vi "Button Grey.vi"(8 "error constant":errorcluster, 9 "Model Name":T1, 10 "appended array 2":bool[](array[boolean]), 11 "appended array":refnum<vi>[](array[refnum])) -> (0 "error constant 2":errorcluster)   [LabVIEW 2017]
uses:
  controls/Model Name.ctl
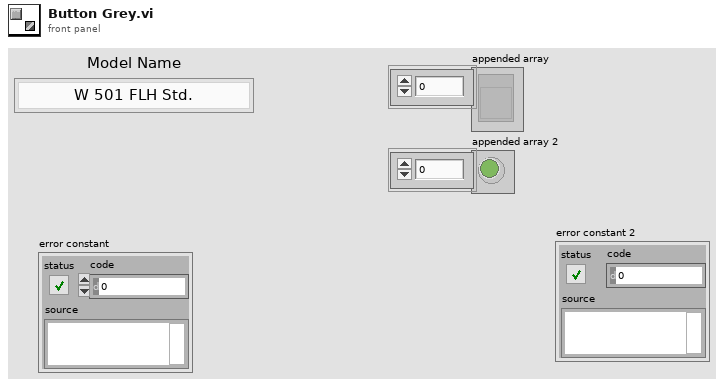
[diagram p1: front panel]
types:
  T1 = typedef "Model Name.ctl" = enum16{"W 501 FLH Std.", "W 501 FRH Std.", "W 601 FR RH Std", "W 601 FR LH Std", "W 601 RR RH Std", "W 601 RR LH Std", "W 601 FR RH AP", "W 601 FR LH AP", "W 601 RR RH AP", "W 601 RR LH AP"}
  T2 = enum8{"Enabled", "Disabled", "Disabled and Grayed Out"}
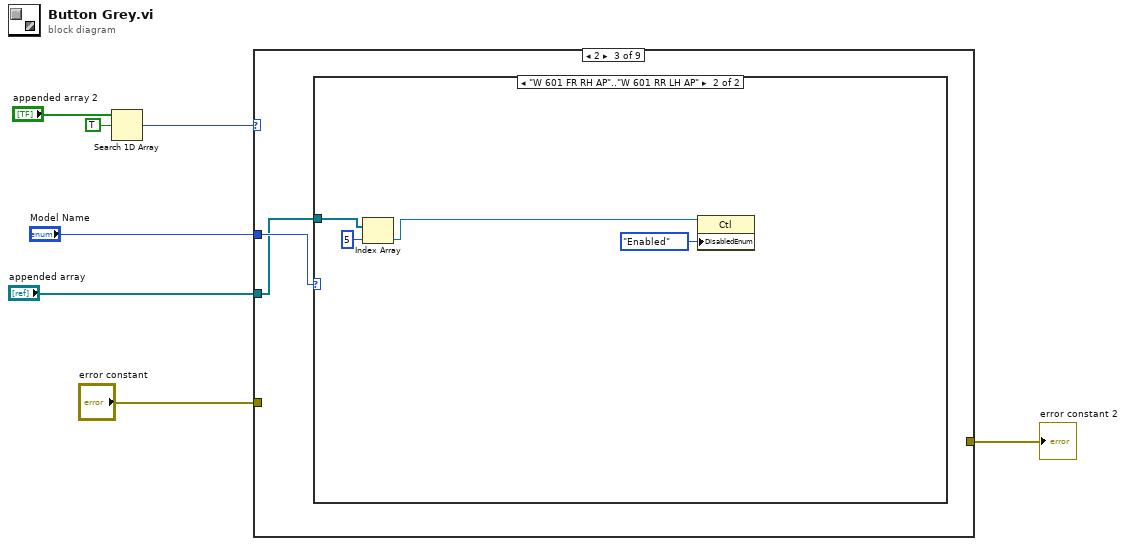
[diagram p0: block diagram]
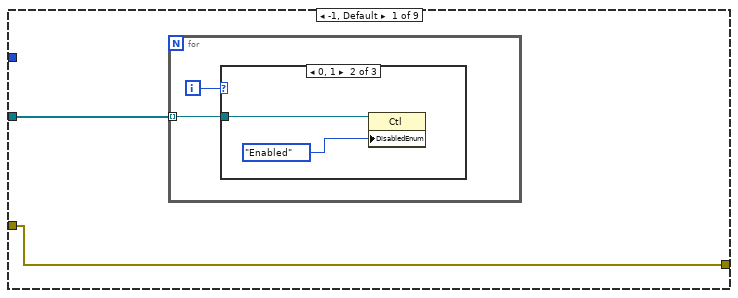
[diagram p2: hidden frame]
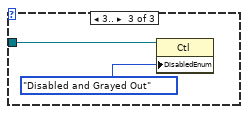
[diagram p4: hidden frame]
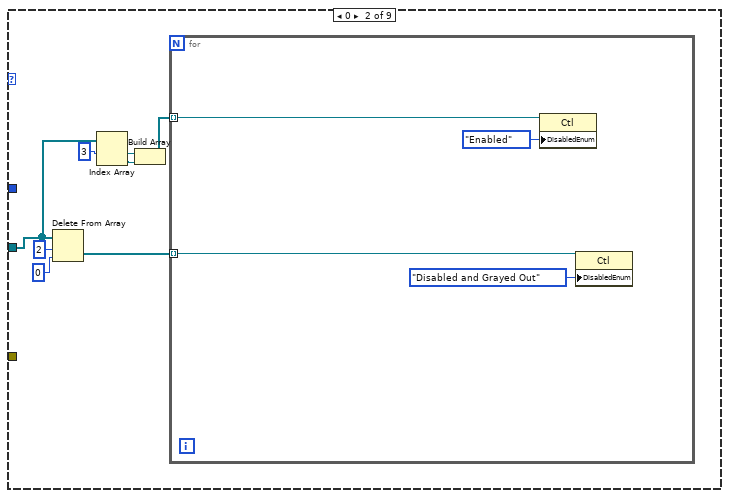
[diagram p5: hidden frame]
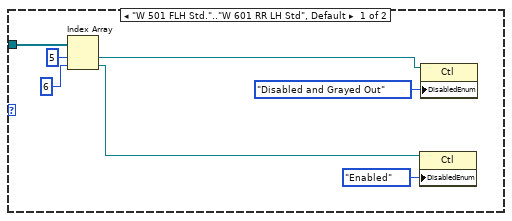
[diagram p6: hidden frame]
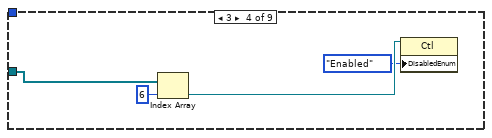
[diagram p7: hidden frame]
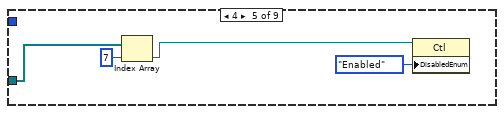
[diagram p8: hidden frame]
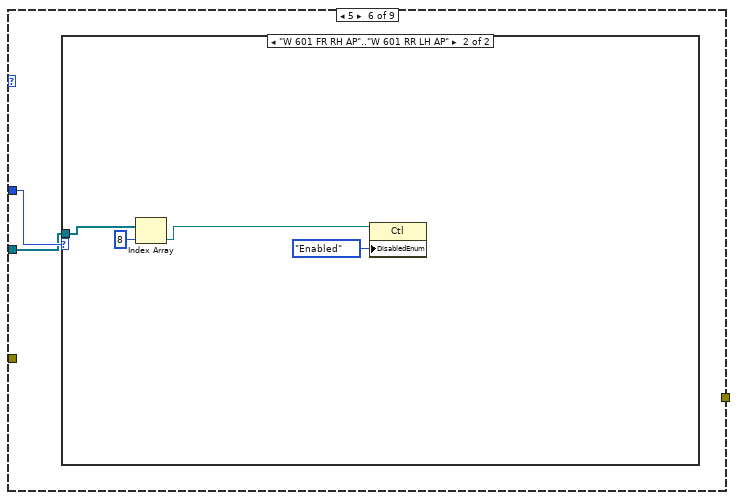
[diagram p9: hidden frame]
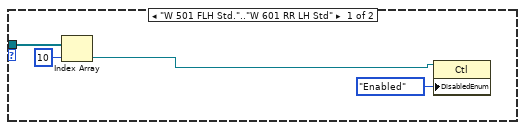
[diagram p10: hidden frame]
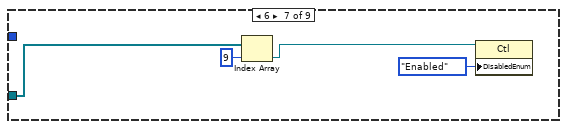
[diagram p11: hidden frame]
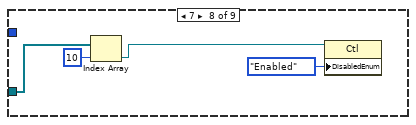
[diagram p12: hidden frame]
diagram:
  n1 = Search 1D Array(1D array="appended array 2", element=TRUE) -> (index of element=w6:i32)  [unwired: 1 in]
  n2 = case shown="2" w6 {
    tunnel: "appended array" -> [w9 w20 w28 w44 w48 w49 w59 w63 _]
    tunnel: "Model Name" -> [_ _ w29 _ _ w50 _ _ _]
    tunnel: "error constant" -> [w8 _ _ _ _ _ _ _ _]
    tunnel: [w8 _ _ _ _ _ _ _ _] -> w1
    frame -1, Default {
      n3 = for {
        tunnel: w9 -> [w10] mode=indexing
        i -> [w11]
        n4 = case shown="0, 1" w11 {
          tunnel: w10 -> [_ w12 w14]
          frame Default {
          }
          frame 0, 1 {
            n5 = property class="Ctl"(reference=w12, "DisabledEnum"=T2."Enabled" ("Disabled")) -> ()  [unwired: 1 in, 2 out]
          }
          frame 3.. {
            n6 = property class="Ctl"(reference=w14, "DisabledEnum"=T2."Disabled and Grayed Out" ("Disabled")) -> ()  [unwired: 1 in, 2 out]
          }
        }
      }
    }
    frame 0 {
      n7 = Delete From Array(array=w20, length=2, index=0) -> (deleted portion=w21:refnum<vi>[])  [unwired: 1 out]
      n8 = Index Array(array=w20, index #1=3 ("index")) -> (element #1=w18:refnum<vi>, element #2=w17:refnum<vi>)  [unwired: 1 in]
      n9 = Build Array(w18, w17) -> (w16:refnum<vi>[])
      n10 = for {
        tunnel: w21 -> [w27] mode=indexing
        tunnel: w16 -> [w25] mode=indexing
        n11 = property class="Ctl"(reference=w25, "DisabledEnum"=T2."Enabled" ("Disabled")) -> ()  [unwired: 1 in, 2 out]
        n12 = property class="Ctl"(reference=w27, "DisabledEnum"=T2."Disabled and Grayed Out" ("Disabled")) -> ()  [unwired: 1 in, 2 out]
      }
    }
    frame 2 {
      n13 = case shown="\"W 601 FR RH AP\"..\"W 601 RR LH AP\"" w29 {
        tunnel: w28 -> [w36 w39]
        frame "W 501 FLH Std.".."W 601 RR LH Std", Default {
          n14 = Index Array(array=w36, index #1=5 ("index"), index #2=6 ("index")) -> (element #1=w35:refnum<vi>, element #2=w34:refnum<vi>)
          n15 = property class="Ctl"(reference=w34, "DisabledEnum"=T2."Enabled" ("Disabled")) -> ()  [unwired: 1 in, 2 out]
          n16 = property class="Ctl"(reference=w35, "DisabledEnum"=T2."Disabled and Grayed Out" ("Disabled")) -> ()  [unwired: 1 in, 2 out]
        }
        frame "W 601 FR RH AP".."W 601 RR LH AP" {
          n17 = Index Array(array=w39, index=5) -> (element=w38:refnum<vi>)
          n18 = property class="Ctl"(reference=w38, "DisabledEnum"=T2."Enabled" ("Disabled")) -> ()  [unwired: 1 in, 2 out]
        }
      }
    }
    frame 3 {
      n19 = Index Array(array=w44, index=6) -> (element=w42:refnum<vi>)
      n20 = property class="Ctl"(reference=w42, "DisabledEnum"=T2."Enabled" ("Disabled")) -> ()  [unwired: 1 in, 2 out]
    }
    frame 4 {
      n21 = Index Array(array=w48, index=7) -> (element=w45:refnum<vi>)
      n22 = property class="Ctl"(reference=w45, "DisabledEnum"=T2."Enabled" ("Disabled")) -> ()  [unwired: 1 in, 2 out]
    }
    frame 5 {
      n23 = case shown="\"W 601 FR RH AP\"..\"W 601 RR LH AP\"" w50 {
        tunnel: w49 -> [w54 w58]
        frame "W 501 FLH Std.".."W 601 RR LH Std" {
          n24 = Index Array(array=w54, index=10) -> (element=w52:refnum<vi>)
          n25 = property class="Ctl"(reference=w52, "DisabledEnum"=T2."Enabled" ("Disabled")) -> ()  [unwired: 1 in, 2 out]
        }
        frame "W 601 FR RH AP".."W 601 RR LH AP" {
          n26 = Index Array(array=w58, index=8) -> (element=w56:refnum<vi>)
          n27 = property class="Ctl"(reference=w56, "DisabledEnum"=T2."Enabled" ("Disabled")) -> ()  [unwired: 1 in, 2 out]
        }
      }
    }
    frame 6 {
      n28 = Index Array(array=w59, index=9) -> (element=w61:refnum<vi>)
      n29 = property class="Ctl"(reference=w61, "DisabledEnum"=T2."Enabled" ("Disabled")) -> ()  [unwired: 1 in, 2 out]
    }
    frame 7 {
      n30 = Index Array(array=w63, index=10) -> (element=w65:refnum<vi>)
      n31 = property class="Ctl"(reference=w65, "DisabledEnum"=T2."Enabled" ("Disabled")) -> ()  [unwired: 1 in, 2 out]
    }
    frame 8 {
    }
  }
  "error constant 2" <- w1
